vi "Eurotherm - Validate Checksum.vi"(7 "Reply":string) -> (8 "Checksum Valid":bool)   [LabVIEW 2011]
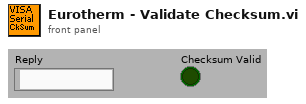
[diagram p1: front panel]
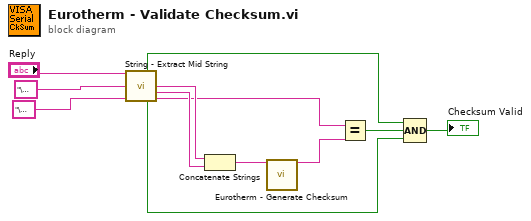
[diagram p0: block diagram]
diagram:
  n1 = call "String - Extract Mid String.vi"("String"="Reply", "Start search string"="\u0002", "End search string"="\u0003") -> ("Start String Found"=w6:bool, "String - Middle"=w9:string, "String - End"=w8:string, "End String Found"=w5:bool, "String - After"=w7:string)  [unwired: 6 in, 2 out]
  n2 = Concatenate Strings(w9, w8) -> (w2:string)
  n3 = call "Eurotherm - Generate Checksum.vi"("String"=w2) -> ("Checksum Character"=w1:string)  [unwired: 13 in, 1 out]
  n4 = Equal?(x=w7, y=w1) -> (x = y?=w4:bool)
  n5 = Compound Arithmetic op=AND(w6, w4, w5) -> (→"Checksum Valid":bool)
